vi "Remove Attribute.vi"(8 "error in (no error)":errorcluster, 10 "Key":string, 11 "Object in":refnum<class "Object.lvclass">) -> (0 "error out":errorcluster, 3 "Object out":refnum<class "Object.lvclass">)   [LabVIEW 2019, in "HierDAL Library.lvlib" / "Models.lvlib" / "Object.lvclass"]
uses:
  Object.lvclass
  Object.lvclass/Object.ctl
  957755c0-9e78-44da-b493-ca416070fd67.vi
  Attribute Class/Attribute.lvclass
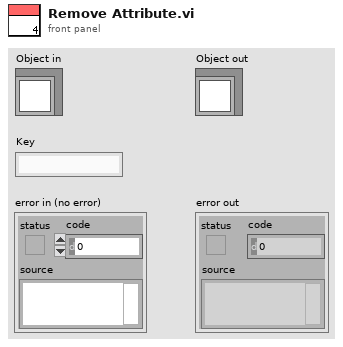
[diagram p1: front panel]
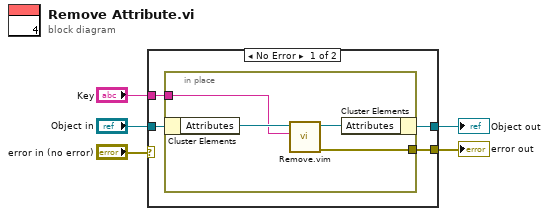
[diagram p0: block diagram]
diagram:
  n1 = case shown="No Error" "error in (no error)" {
    selector: "error in (no error)" -> [_ w15]
    tunnel: [w7 w15] -> w4
    tunnel: [w6 w14] -> w2
    tunnel: "Object in" -> [w9 w14]
    tunnel: "Key" -> [w8 _]
    frame No Error {
      n2 = in-place {
        in-place-border: w8 -> [w12]
        in-place-border: [w10] -> w7
        n3 = in-place-cluster #1(w9) -> ("Attributes"=w13:refnum<data-value>)
        n4 = call "Remove.vim"("Key"=w12, "Map DVR in"=w13) -> ("error out"=w10:errorcluster, "Map DVR out"=w11:refnum<data-value>)  [unwired: 6 in, 2 out]
        n5 = in-place-cluster #1("Attributes"=w11) -> (w6:refnum<class "Object.lvclass">)
      }
    }
    frame Error {
    }
  }
  "error out" <- w4
  "Object out" <- w2
